vi "Read SupportBulkCreate.vi"(8 "error in (no error)":errorcluster, 11 "DbConnection in":refnum<class "DbConnection.lvclass">) -> (0 "error out":errorcluster, 2 "SupportBulkCreate":bool, 3 "DbConnection out":refnum<class "DbConnection.lvclass">)   [LabVIEW 2020, in "ORM.lvlib" / "DbConnection.lvclass"]
uses:
  DbConnection.lvclass
  DbConnection.lvclass/DbConnection.ctl
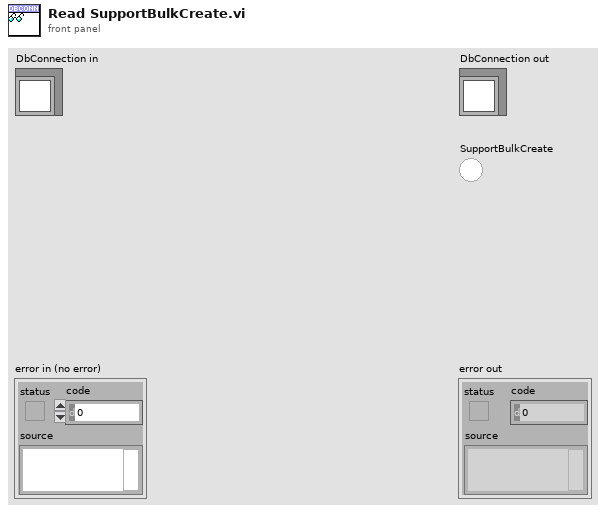
[diagram p1: front panel]
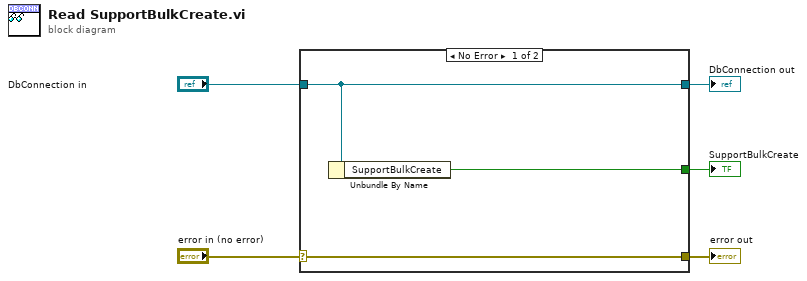
[diagram p0: block diagram]
diagram:
  n1 = case shown="No Error" "error in (no error)" {
    selector: "error in (no error)" -> [w8 w9]
    tunnel: [w8 w9] -> w4
    tunnel: [w7 w10] -> w2
    tunnel: "DbConnection in" -> [w7 w10]
    tunnel: [w6 _] -> w1
    frame No Error {
      n2 = Unbundle By Name(w7) -> ("SupportBulkCreate"=w6:bool)
    }
    frame Error {
    }
  }
  "error out" <- w4
  "DbConnection out" <- w2
  "SupportBulkCreate" <- w1
